vi "Update Fan Status.vi"(8 "error in (no error)":errorcluster, 9 "Fan B":T1, 10 "Fan A":T1, 11 "Evaporative Cooler":refnum<class "Evaporative Cooler.lvclass">) -> (0 "error out":errorcluster, 3 "Evaporative Cooler":refnum<class "Evaporative Cooler.lvclass">)   [LabVIEW 2018, in "Evaporative Cooler.lvlib" / "Evaporative Cooler.lvclass"]
doc: "This method sends a message to the controller letting it know information about both of the fans."
uses:
  Evaporative Cooler/Evaporative Cooler/Evaporative Cooler.lvclass
  C:/GitClones/LGP5-Resources/Frameworks/Actor Framework/Feedback Evaporative Cooler/Cooler/Cooler/Cooler.lvclass
  Dual Fan/Dual Fan/Fan Info.ctl
  <vilib>/ActorFramework/Message Enqueuer/Message Enqueuer.lvclass
  Cooler.lvclass/Cooler.ctl
  Evaporative Cooler Controller/Update Fan Status Msg/Update Fan Status Msg.lvclass/Update Fan Status Msg.ctl
  <vilib>/ActorFramework/Message Enqueuer/Message Enqueuer.lvclass/Message Enqueuer.ctl
  <vilib>/ActorFramework/Message Enqueuer/Enqueue.vi
  Evaporative Cooler Controller/Update Fan Status Msg/Update Fan Status Msg.lvclass
  C:/Program Files (x86)/National Instruments/LabVIEW 2018/vi.lib/ActorFramework/Message/Message.lvclass
  <vilib>/ActorFramework/Message Priority Queue/Priority Enqueue.vi
  Cooler.lvclass
  Dual Fan/Dual Fan/Dual Fan.lvclass
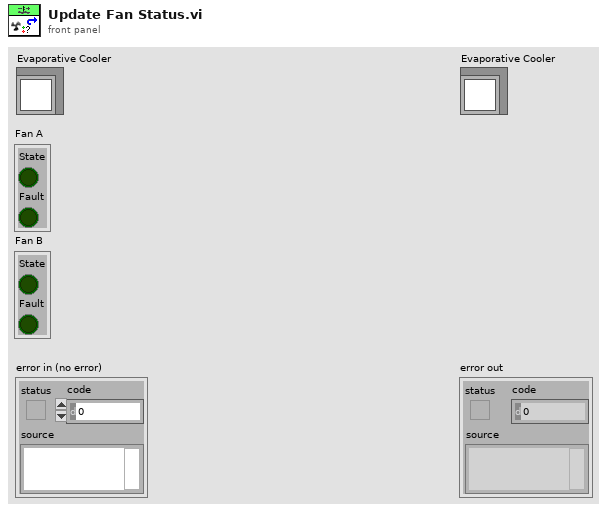
[diagram p1: front panel]
types:
  T1 = typedef "Dual Fan.lvlib/Dual Fan.lvclass/Fan Info.ctl" = cluster{"State":bool, "Fault":bool}
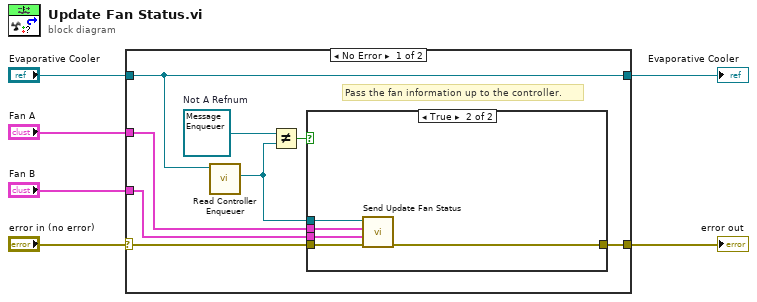
[diagram p0: block diagram]
diagram:
  n1 = case shown="No Error" "error in (no error)" {
    selector: "error in (no error)" -> [w11 w22]
    tunnel: [w10 w22] -> w5
    tunnel: [w14 w21] -> w3
    tunnel: "Evaporative Cooler" -> [w14 w21]
    tunnel: "Fan A" -> [w13 _]
    tunnel: "Fan B" -> [w12 _]
    frame No Error {
      w8 = refnum<class "Message Enqueuer.lvclass"> refnum  # Not A Refnum
      # "Pass the fan information up to the controller."
      n2 = call "Read Controller Enqueuer.vi"("Cooler"=w14) -> ("Controller Enqueuer"=w9:refnum<class "Message Enqueuer.lvclass">)  [unwired: 10 in]
      n3 = Not Equal?(x=w8, y=w9) -> (x != y?=w7:bool)
      n4 = case shown="True" w7 {
        tunnel: w9 -> [_ w20]
        tunnel: w13 -> [_ w19]
        tunnel: w12 -> [_ w18]
        tunnel: w11 -> [w15 w17]
        tunnel: [w15 w16] -> w10
        frame False {
        }
        frame True {
          n5 = call "Send Update Fan Status.vi"("error in (no error)"=w17, "Fan B"=w18, "Fan A"=w19, "Message Enqueuer"=w20) -> ("error out"=w16:errorcluster)  [unwired: 7 in]
        }
      }
    }
    frame Error {
    }
  }
  "error out" <- w5
  "Evaporative Cooler" <- w3
